vi "Regenerate Linker Cache.vi"() -> ()   [LabVIEW 2019, in "HawkeyeToolsMenu.lvlib"]
doc: "GUI to compare LabVIEW code between currently checked out branch with any other branch or any of its commits.\n\n(c) 2024 Soliton Technologies. All rights reserved."
uses:
  HawkeyeToolsMenu.lvlib
  <userlib>/_OpenG.lib/file/file.llb/File Exists - Scalar__ogtk.vi
  <userlib>/_OpenG.lib/file/file.llb/Valid Path - Traditional__ogtk.vi
  vi.lib/Hawkeye/Hawkeye.lvlib
panel:
  in  "Tab Control":enum32{"Main UI", "About"}(tab)
  out "Current Status":string
  in  "Stop":bool
  in  "Repo / Workspace Folder Path":path
  in  "Regenerate":bool
  # "This GUI allows you to regenerate Linker Cache lists for the entire repository ensuring Linker information is up to date."
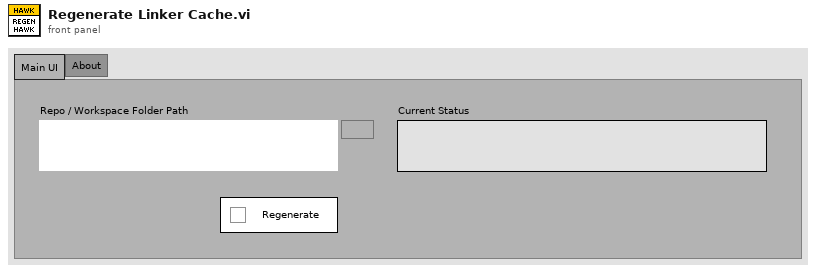
[diagram p1: front panel]
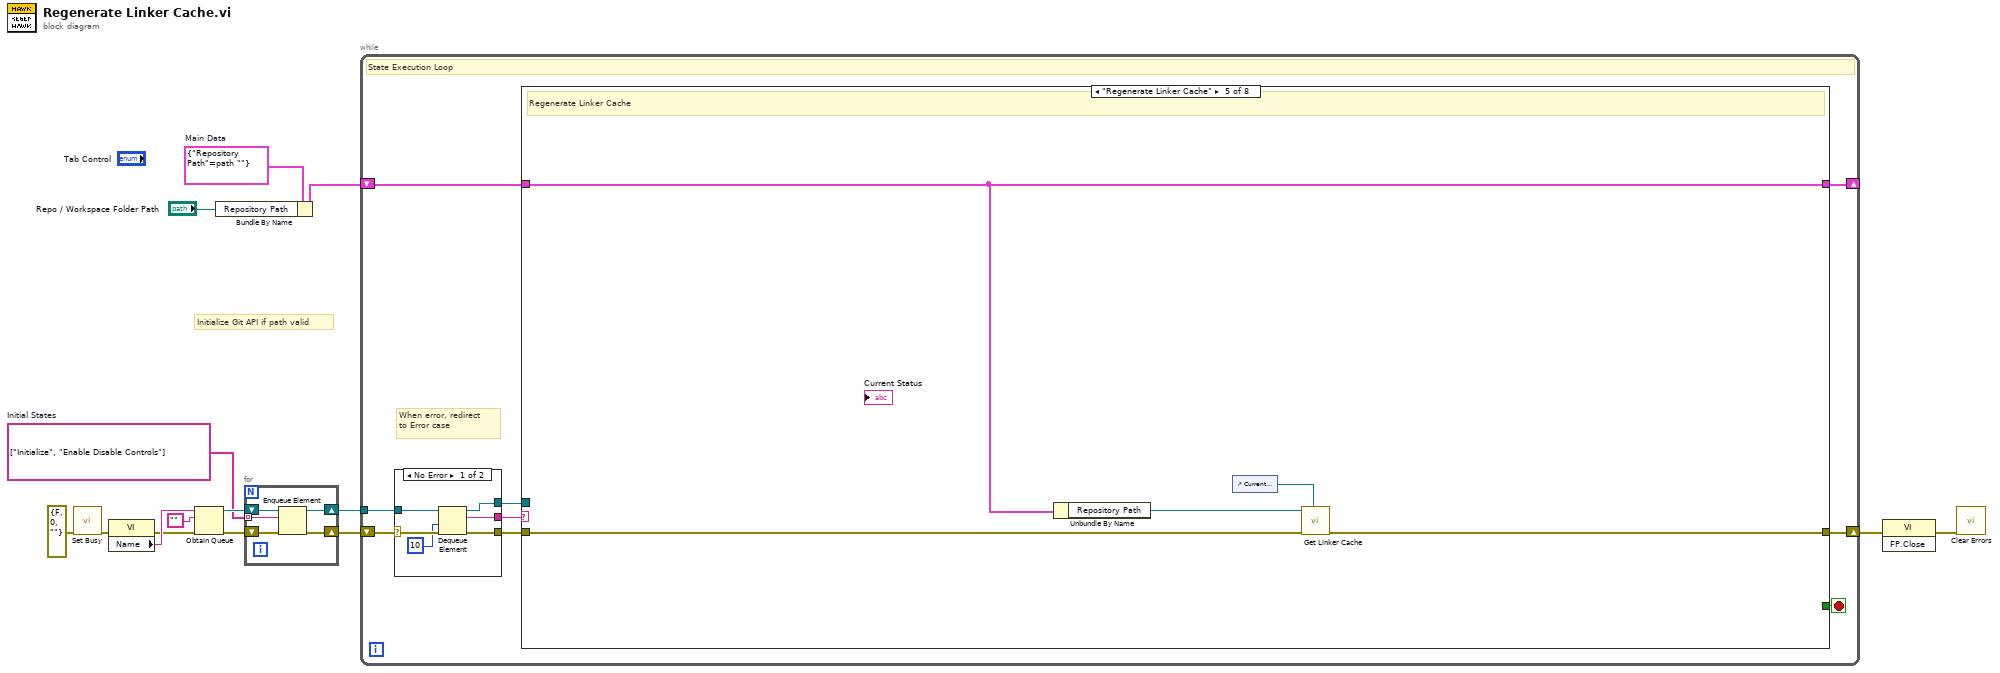
[diagram p0: block diagram]
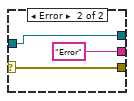
[diagram p2: hidden frame]
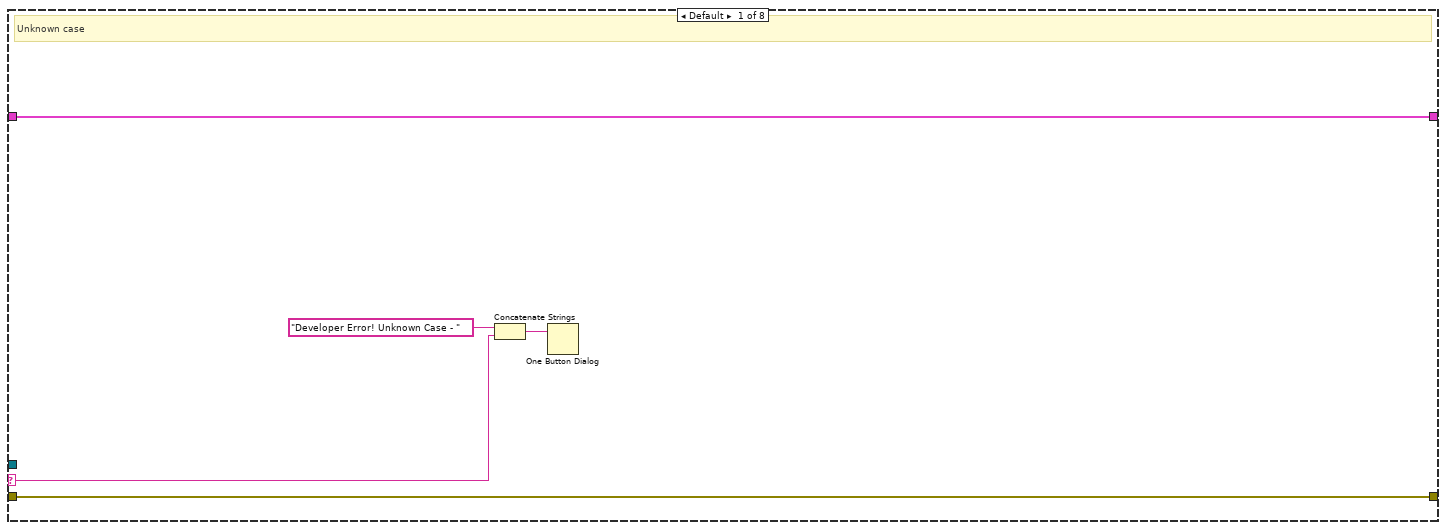
[diagram p3: hidden frame]
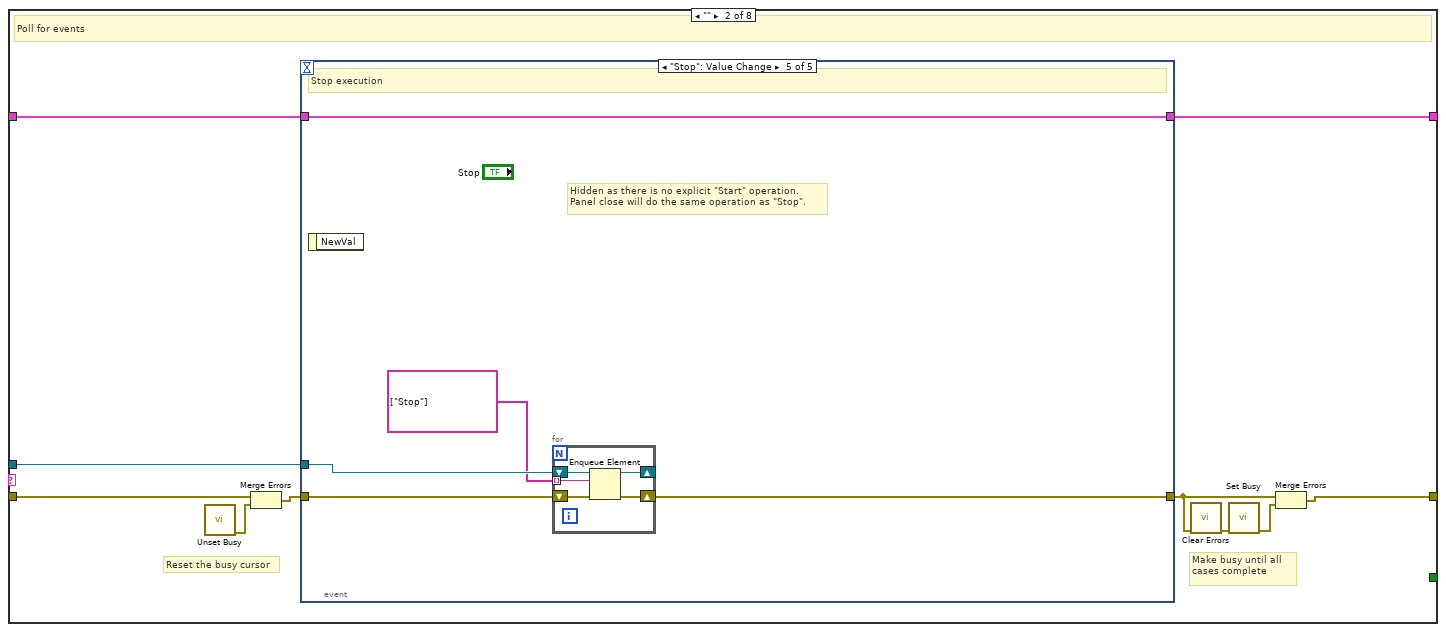
[diagram p4: hidden frame]
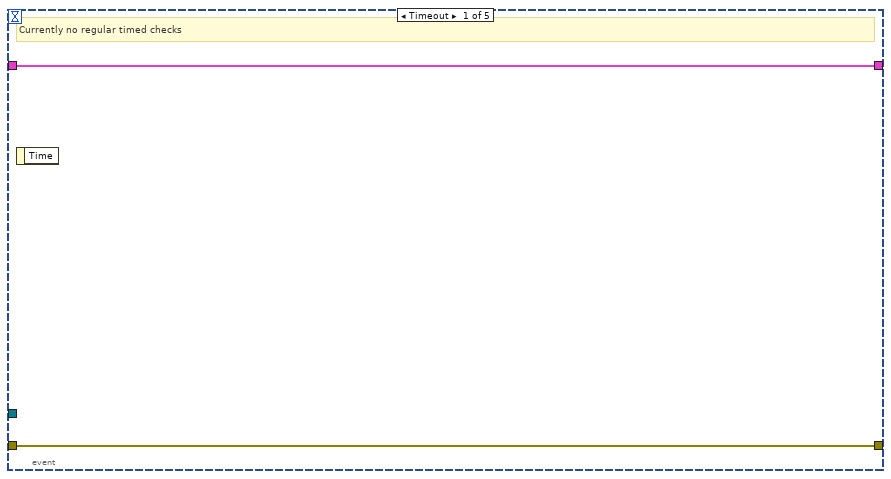
[diagram p5: hidden frame]
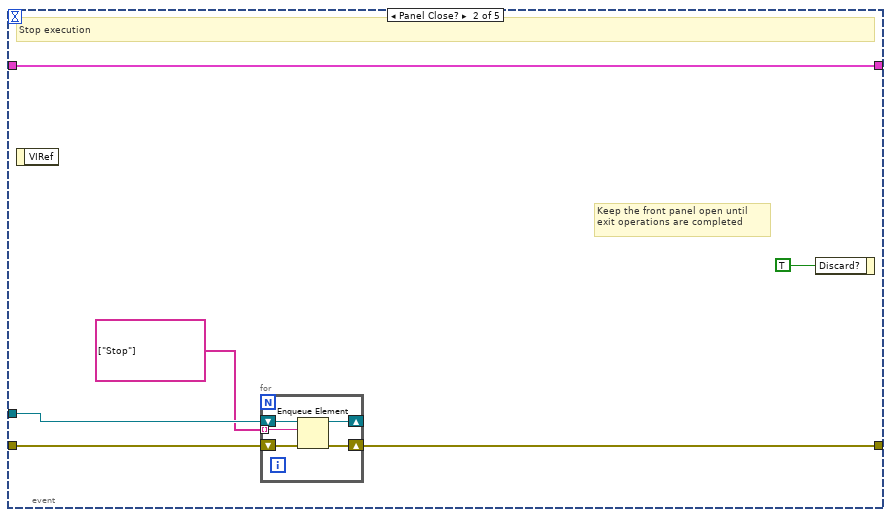
[diagram p6: hidden frame]
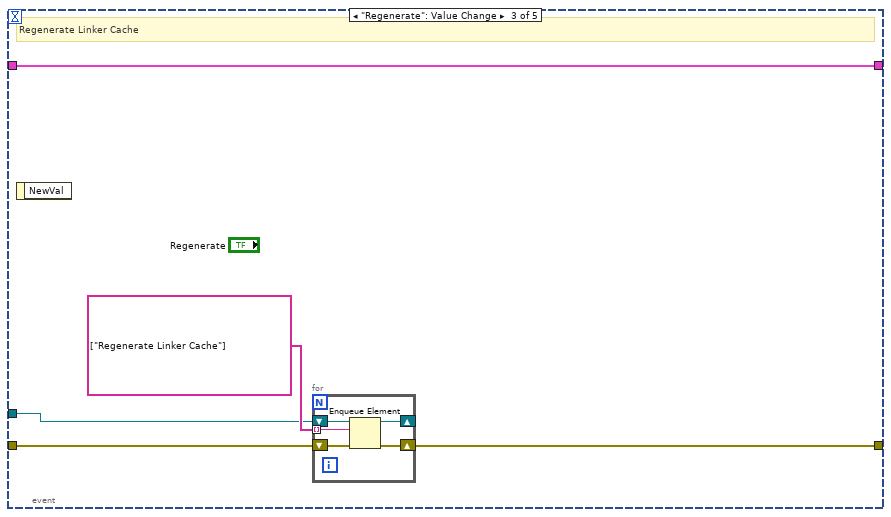
[diagram p7: hidden frame]
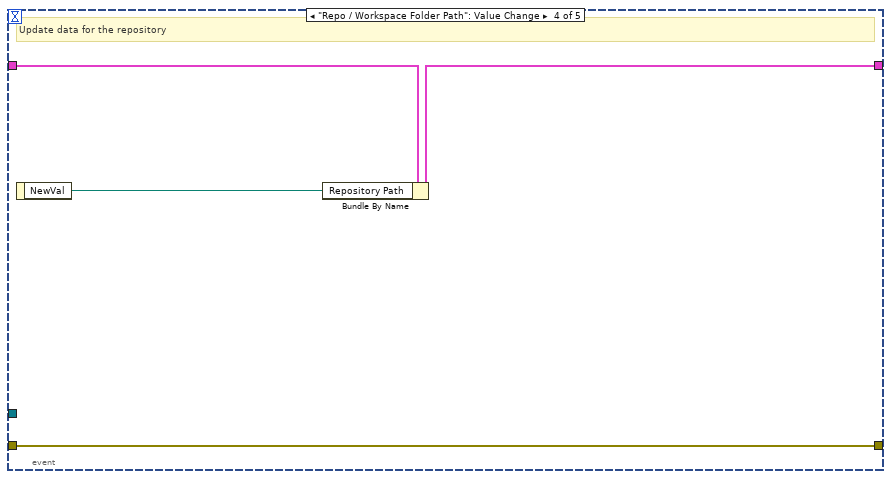
[diagram p8: hidden frame]
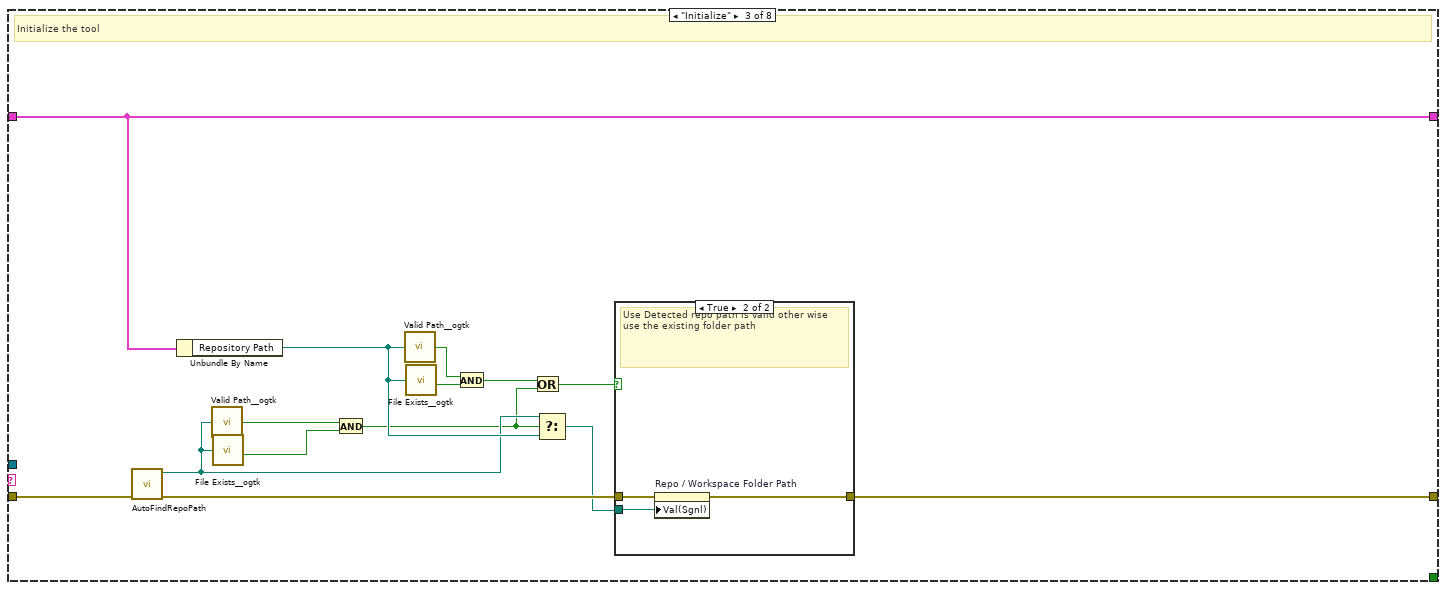
[diagram p9: hidden frame]
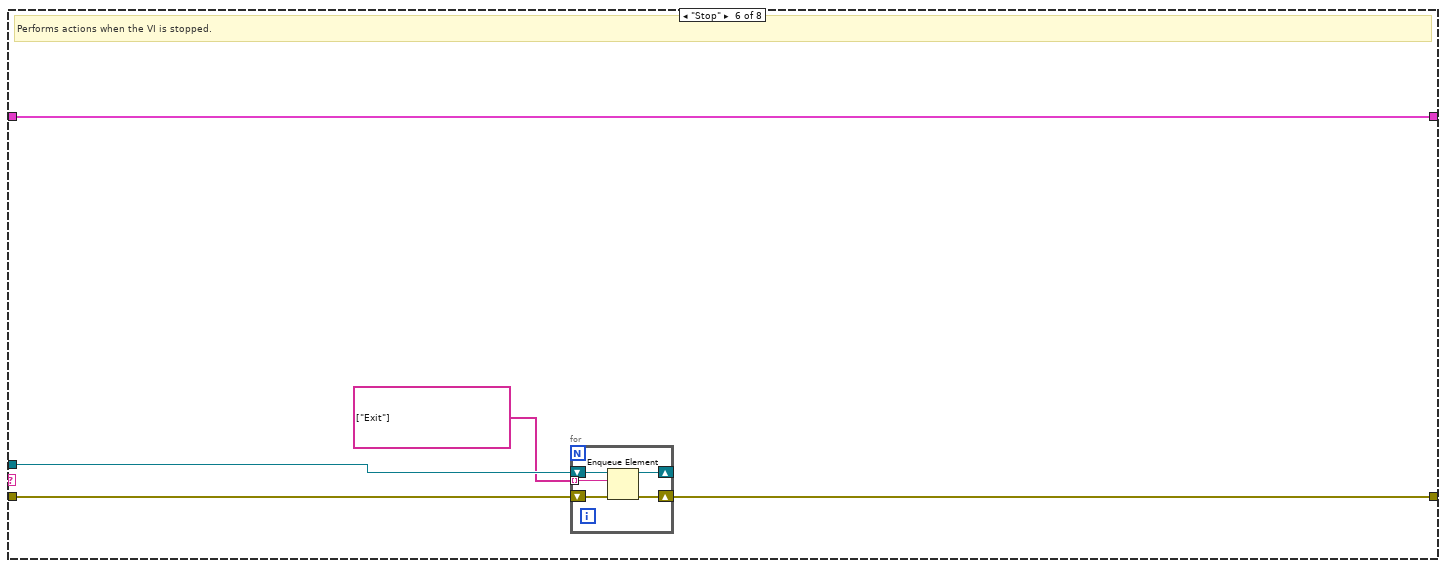
[diagram p12: hidden frame]
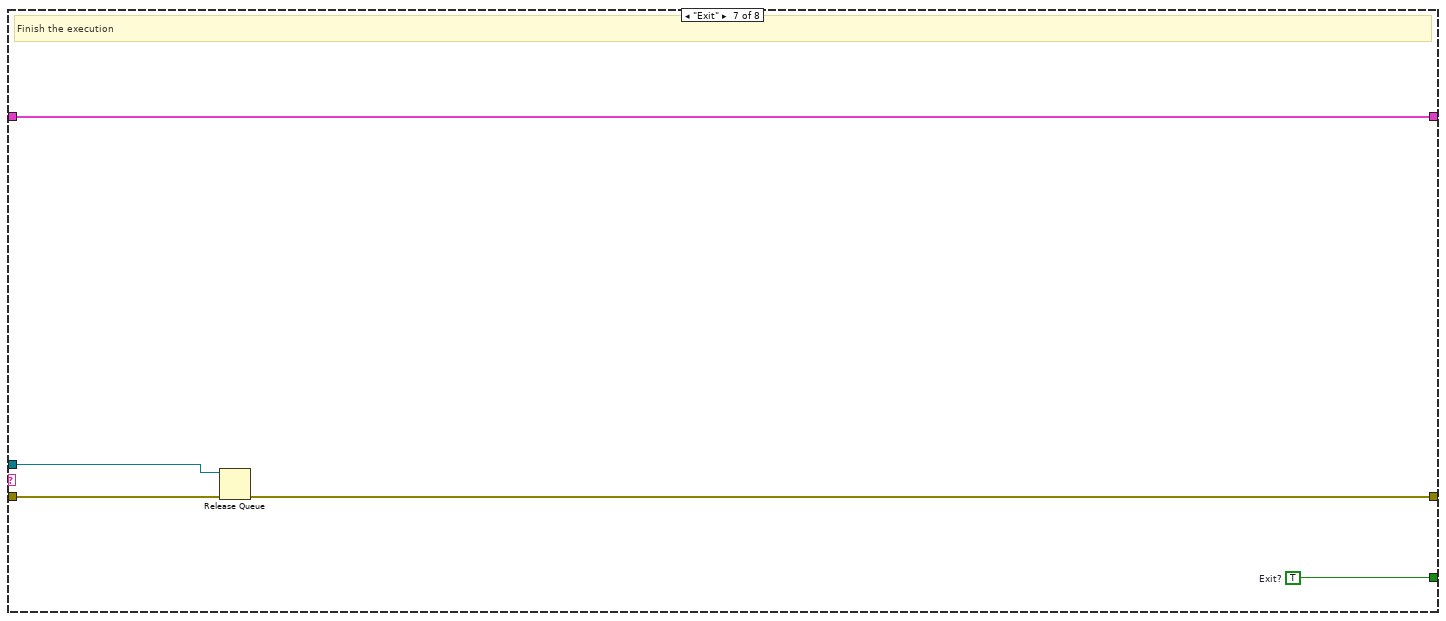
[diagram p13: hidden frame]
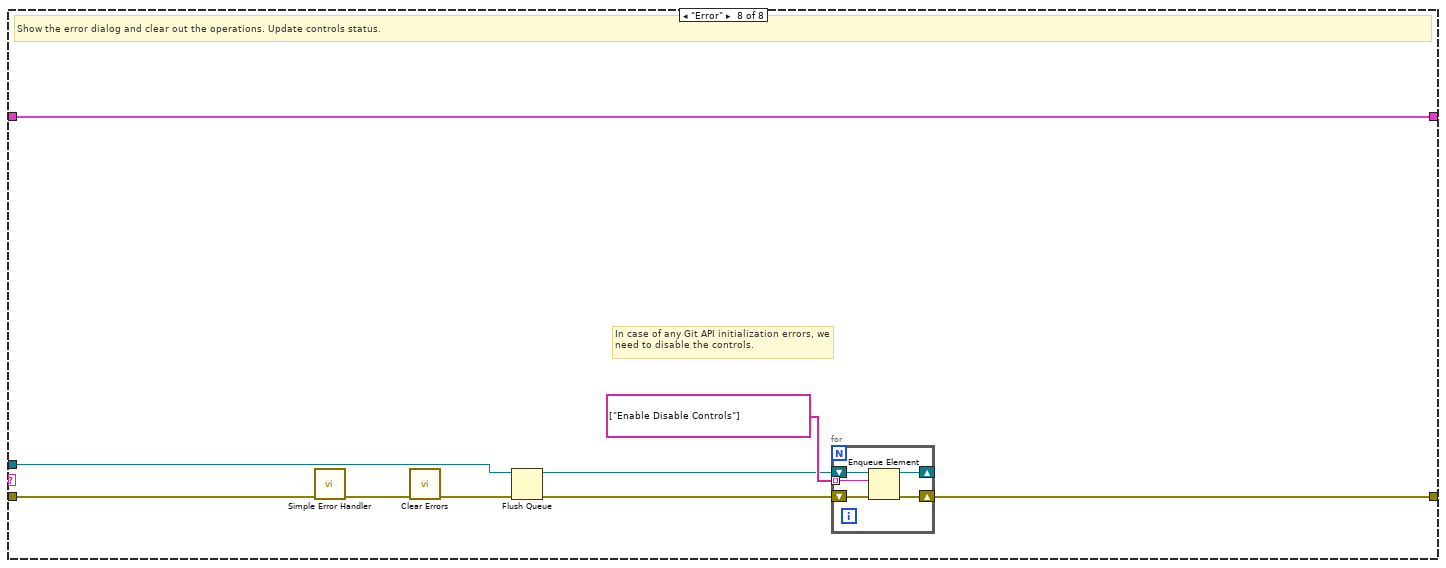
[diagram p14: hidden frame]
diagram:
  w1 = string[] ["Initialize", "Enable Disable Controls"]  # Initial States
  w12 = cluster{"Repository Path":path} {"Repository Path"=path ""}  # Main Data
  # "Initialize Git API if path valid"
  n1 = call <vilib>:"Set Busy.vi"("error in (no error)"=errorcluster {"status"=FALSE, "code"=0, "source"=""}) -> ("error out"=w5:errorcluster)  [unwired: 9 in, 1 out]
  n2 = property class="VI"(error in=w5) -> (error out=w14:errorcluster, "Name"=w15:string)  [unwired: 1 in, 1 out]
  n3 = Obtain Queue(name (unnamed)=w15, element data type="", error in (no error)=w14) -> (queue out=w10:refnum<queue>, error out=w7:errorcluster)  [unwired: 2 in, 1 out]
  n4 = Bundle By Name(cluster=w12, "Repository Path"="Repo / Workspace Folder Path") -> (w11:cluster{"Repository Path":path})
  n5 = for {
    tunnel: w1 -> [w17] mode=indexing
    shift-right: [w19] -> w9
    shift-left: w7 -> [w20]
    shift-right: [w16] -> w8
    shift-left: w10 -> [w18]
    n6 = Enqueue Element(queue=w18, element=w17, error in (no error)=w20) -> (queue out=w16:refnum<queue>, error out=w19:errorcluster)  [unwired: 1 in, 1 out]
  }
  n7 = while {
    shift-right: [w21] -> w3
    shift-left: w9 -> [w23]
    tunnel: w8 -> [w24]
    shift-right: [w26] -> _
    shift-left: w11 -> [w25]
    stop <- w27 stop-if-true
    # "When error, redirect to Error case"
    # "State Execution Loop"
    n8 = case shown="No Error" w23 {
      selector: w23 -> [w32 w36]
      tunnel: [w35 "Error" ("element")] -> w29
      tunnel: [w34 w38] -> w28
      tunnel: w24 -> [w33 w38]
      tunnel: [w30 w36] -> w22
      frame No Error {
        n9 = Dequeue Element(queue=w33, timeout in ms (-1)=10, error in (no error)=w32) -> (queue out=w34:refnum<queue>, element=w35:string, error out=w30:errorcluster)  [unwired: 1 out]
      }
      frame Error {
      }
    }
    n10 = case shown="\"Regenerate Linker Cache\"" w29 {
      selector: w29 -> [w42 _ _ _ _ _ _ _]
      tunnel: w22 -> [w40 w47 w103 w109 w114 w120 w130 w138]
      tunnel: w28 -> [_ w53 _ _ _ w118 w127 w135]
      tunnel: [w40 w49 w91 w109 w111 w119 w126 w131] -> w21
      tunnel: [_ _ _ _ _ _ w128 _] -> w27
      tunnel: [w39 w51 w100 w110 w115 w117 w129 w139] -> w26
      tunnel: w25 -> [w39 w52 w100 w110 w115 w117 w129 w139]
      frame Default {
        # "Unknown case"
        n11 = Concatenate Strings("Developer Error! Unknown Case - " ("string"), w42) -> (w41:string)
        n12 = One Button Dialog(message=w41) -> ()  [unwired: 1 in, 1 out]
      }
      frame "" {
        # "Reset the busy cursor"
        # "Make busy until all cases complete"
        # "Poll for events"
        n13 = call <vilib>:"Unset Busy.vi"() -> ("error out"=w48:errorcluster)  [unwired: 11 in]
        n14 = Merge Errors(w47, w48) -> (w46:errorcluster)
        n15 = event shown="[4] \"Stop\": Value Change" {
          selector: _ -> [_ _ _ _ _]
          dyn-events: _ -> [_ _ _ _ _]
          timeout: _ -> [_ _ _ _ _]
          tunnel: w46 -> [w54 w61 w70 w77 w85]
          tunnel: w53 -> [_ w60 w69 _ w84]
          tunnel: [w54 w59 w68 w77 w83] -> w45
          tunnel: w52 -> [w55 w58 w67 w80 w82]
          tunnel: [w55 w58 w67 w79 w82] -> w51
          event Timeout {
            # "Currently no regular timed checks"
            n16 = event-data() -> ()  [unwired: 1 in, 1 out]
          }
          event Panel Close? {
            # "Keep the front panel open until exit operations are completed"
            # "Stop execution"
            n17 = event-data() -> ()  [unwired: 1 in, 1 out]
            n18 = for {
              tunnel: string[] ["Stop"] -> [w63] mode=indexing
              shift-right: [w65] -> w59
              shift-left: w61 -> [w66]
              shift-right: [w62] -> _
              shift-left: w60 -> [w64]
              n19 = Enqueue Element(queue=w64, element=w63, error in (no error)=w66) -> (queue out=w62:refnum<queue>, error out=w65:errorcluster)  [unwired: 1 in, 1 out]
            }
            n20 = event-data("Discard?"=TRUE) -> ()  [unwired: 1 in, 1 out]
          }
          event "Regenerate": Value Change {
            # "Regenerate Linker Cache"
            n21 = event-data() -> ()  [unwired: 1 in, 1 out]
            n22 = for {
              tunnel: string[] ["Regenerate Linker Cache"] -> [w73] mode=indexing
              shift-right: [w75] -> w68
              shift-left: w70 -> [w76]
              shift-right: [w72] -> _
              shift-left: w69 -> [w74]
              n23 = Enqueue Element(queue=w74, element=w73, error in (no error)=w76) -> (queue out=w72:refnum<queue>, error out=w75:errorcluster)  [unwired: 1 in, 1 out]
            }
          }
          event "Repo / Workspace Folder Path": Value Change {
            # "Update data for the repository"
            n24 = event-data() -> ("NewVal"=w78:path)  [unwired: 1 in]
            n25 = Bundle By Name(cluster=w80, "Repository Path"=w78) -> (w79:cluster{"Repository Path":path})
          }
          event "Stop": Value Change {
            # "Hidden as there is no explicit \"Start\" operation.\nPanel close will do the same operation as \"Stop\"."
            # "Stop execution"
            n26 = event-data() -> ()  [unwired: 1 in, 1 out]
            n27 = for {
              tunnel: string[] ["Stop"] -> [w87] mode=indexing
              shift-right: [w89] -> w83
              shift-left: w85 -> [w90]
              shift-right: [w86] -> _
              shift-left: w84 -> [w88]
              n28 = Enqueue Element(queue=w88, element=w87, error in (no error)=w90) -> (queue out=w86:refnum<queue>, error out=w89:errorcluster)  [unwired: 1 in, 1 out]
            }
          }
        }
        n29 = call <vilib>:"Clear Errors.vi"("error in (no error)"=w45) -> ("error out"=w44:errorcluster)  [unwired: 5 in, 1 out]
        n30 = call <vilib>:"Set Busy.vi"("error in (no error)"=w44) -> ("error out"=w50:errorcluster)  [unwired: 9 in, 1 out]
        n31 = Merge Errors(w45, w50) -> (w49:errorcluster)
      }
      frame "Initialize" {
        # "Initialize the tool"
        n32 = call "AutoFindRepoPath.vi"("error in (no error)"=w103) -> ("error out"=w104:errorcluster, "Repo Path"=w94:path)  [unwired: 9 in]
        n33 = Unbundle By Name(w100) -> ("Repository Path"=w96:path)
        n34 = call-poly <userlib>:"Valid Path__ogtk.vi"("path"=w94) -> ("valid"=w101:bool)
        n35 = call-poly <userlib>:"File Exists__ogtk.vi"("file path"=w94) -> ("exists"=w102:bool)  [unwired: 6 in, 1 out]
        n36 = And(x=w101, y=w102) -> (x .and. y?=w93:bool)
        n37 = call-poly <userlib>:"Valid Path__ogtk.vi"("path"=w96) -> ("valid"=w95:bool)
        n38 = call-poly <userlib>:"File Exists__ogtk.vi"("file path"=w96) -> ("exists"=w99:bool)  [unwired: 6 in, 1 out]
        n39 = And(x=w95, y=w99) -> (x .and. y?=w98:bool)
        n40 = Or(x=w98, y=w93) -> (x .or. y?=w97:bool)
        n41 = Select(t=w94, s=w93, f=w96) -> (s? t:f=w92:path)
        n42 = case shown="True" w97 {
          tunnel: w104 -> [w105 w108]
          tunnel: [w105 w106] -> w91
          tunnel: w92 -> [_ w107]
          frame False {
          }
          frame True {
            # "Use Detected repo path is valid other wise use the existing folder path"
            n43 = property on="Repo / Workspace Folder Path" class="Path"(error in=w108, "Val(Sgnl)"=w107) -> (error out=w106:errorcluster)  [unwired: 1 in, 1 out]
          }
        }
      }
      frame "Enable Disable Controls" {
        # "Not in Use"
        # "Enable or disable controls based on Git API initialized or not"
      }
      frame "Regenerate Linker Cache" {
        # "Regenerate Linker Cache"
        n44 = Unbundle By Name(w115) -> ("Repository Path"=w113:path)
        n45 = control-ref of="Current Status"() -> (w112:refnum<vi>)
        n46 = call "Get Linker Cache.vi"("Status Ref"=w112, "error in (no error)"=w114, "WorkSpace / Repo path"=w113) -> ("error out"=w111:errorcluster)  [unwired: 5 in, 3 out]
      }
      frame "Stop" {
        # "Performs actions when the VI is stopped."
        n47 = for {
          tunnel: string[] ["Exit"] -> [w122] mode=indexing
          shift-right: [w124] -> w119
          shift-left: w120 -> [w125]
          shift-right: [w121] -> _
          shift-left: w118 -> [w123]
          n48 = Enqueue Element(queue=w123, element=w122, error in (no error)=w125) -> (queue out=w121:refnum<queue>, error out=w124:errorcluster)  [unwired: 1 in, 1 out]
        }
      }
      frame "Exit" {
        w128 = TRUE  # Exit?
        # "Finish the execution"
        n49 = Release Queue(queue=w127, error in (no error)=w130) -> (error out=w126:errorcluster)  [unwired: 1 in, 2 out]
      }
      frame "Error" {
        # "In case of any Git API initialization errors, we need to disable the controls."
        # "Show the error dialog and clear out the operations. Update controls status."
        n50 = call <vilib>:"Simple Error Handler.vi"("error in (no error)"=w138) -> ("error out"=w137:errorcluster)  [unwired: 4 in, 4 out]
        n51 = call <vilib>:"Clear Errors.vi"("error in (no error)"=w137) -> ("error out"=w136:errorcluster)  [unwired: 5 in, 1 out]
        n52 = Flush Queue(queue=w135, error in (no error)=w136) -> (queue out=w132:refnum<queue>, error out=w133:errorcluster)  [unwired: 1 out]
        n53 = for {
          tunnel: string[] ["Enable Disable Controls"] -> [w141] mode=indexing
          shift-right: [w143] -> w131
          shift-left: w133 -> [w144]
          shift-right: [w140] -> _
          shift-left: w132 -> [w142]
          n54 = Enqueue Element(queue=w142, element=w141, error in (no error)=w144) -> (queue out=w140:refnum<queue>, error out=w143:errorcluster)  [unwired: 1 in, 1 out]
        }
      }
    }
  }
  n55 = invoke class="VI" method="FP.Close"(error in=w3) -> (error out=w2:errorcluster)  [unwired: 2 in, 2 out]
  n56 = call <vilib>:"Clear Errors.vi"("error in (no error)"=w2) -> ()  [unwired: 5 in, 2 out]
